vi "QueryServer_AddQueryEvent.vi"(11 "gRPCid in":T1) -> (2 "QueryServer_Query":refnum<user-event>, 3 "gRPCid":T1)   [LabVIEW 2019, in "labview-grpc-query-server.lvlib"]
uses:
  labview-grpc-query-server.lvlib
  QueryServer_InvokeEventData.ctl
  gRPC interface/Server API/typeDefs/grpcId.ctl
  QueryServer_QueryEventData.ctl
  a66ee327-264b-4784-bac1-fff8ba4a2692.vi
  gRPC interface/gprc-lvsupport.lvlib
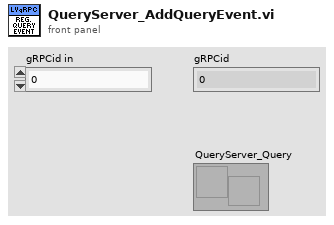
[diagram p1: front panel]
types:
  T1 = typedef "gprc-lvsupport.lvlib/grpcId.ctl" = u64
  T2 = typedef "labview-grpc-query-server.lvlib/QueryServer_QueryEventData.ctl" = cluster{"gRPCid":T1}
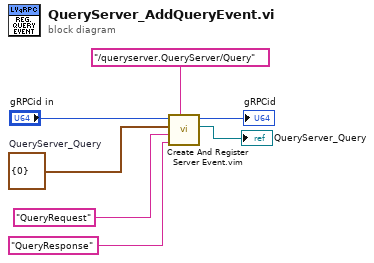
[diagram p0: block diagram]
diagram:
  w5 = T2 {"gRPCid"=0}  # QueryServer_Query
  n1 = call "Create And Register Server Event.vim"("Method name"="/queryserver.QueryServer/Query" ("name"), "Response Metadata Name"="QueryResponse" ("Name"), "Request Metadata Name"="QueryRequest" ("Name"), "event in"=w5, "gRPCid server in"="gRPCid in") -> ("event"=→"QueryServer_Query":refnum<user-event>, "gRPCid server out"=→"gRPCid":T1)  [unwired: 4 in, 1 out]
